vi "Enqueue MHL Queue-single.vi"(7 "Add To Front (F)":bool, 8 "ErrorIn":errorcluster, 10 "Data":variant, 11 "Command":string) -> (0 "ErrorOut":errorcluster)   [LabVIEW 2020, in "main.lvlib"]
doc: "Enqueue to MHL Queue"
uses:
  main.lvlib
  PTRL/QueueHandler/SubVis/Write.vi
  PTRL/QueueHandler/QueueHandler.lvlib
panel:
  # "Description\n\nEnqueue to MHL Queue"
  # "INPUTS"
  # "OUTPUTS"
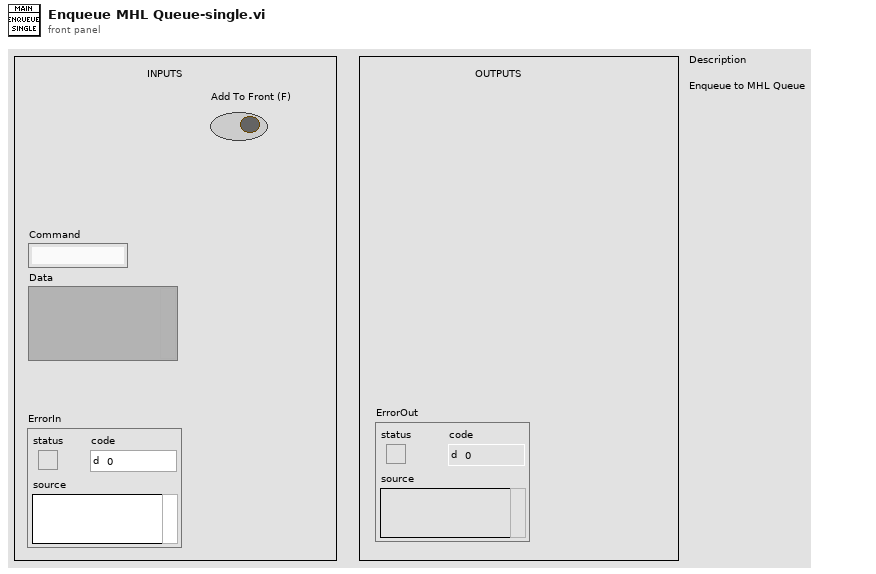
[diagram p1: front panel]
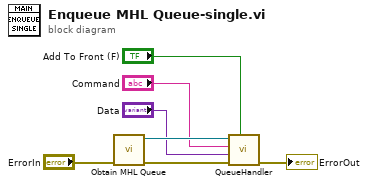
[diagram p0: block diagram]
diagram:
  n1 = call "Obtain MHL Queue.vi"("ErrorIn"="ErrorIn") -> ("ErrorOut"=w2:errorcluster, "MHL Queue Out"=w5:refnum<queue>)  [unwired: 9 in]
  n2 = call-poly "QueueHandler.vi"("AddToFront(F)"="Add To Front (F)", "ErrorIn"=w2, "Data"="Data", "Command"="Command", "MHL Queue In"=w5) -> ("ErrorOut"=→"ErrorOut":errorcluster)  [unwired: 4 in, 2 out]
